vi "Get Dependent Modules.vi"(8 "error in (no error)":errorcluster, 11 "Routing and Faulting Ref in":T1 format="%.0x") -> (0 "error out":errorcluster, 2 "Dependent Modules":T2(array[cluster]) {"Module Ref" format="%.0x"}, 3 "Routing and Faulting Ref out":T1 format="%.0x")   [LabVIEW 2017, in "Routing and Faulting System Explorer.lvlib"]
uses:
  Routing and Faulting System Explorer.lvlib
  <vilib>/NI Veristand/Custom Device API/Custom Device Item Ref.ctl
  <vilib>/NI Veristand/Custom Device API/Get Item Property (String Array).vi
  <vilib>/NI Veristand/Custom Device API/Get Item Property (Dependent Node Pointer).vi
  <vilib>/NI Veristand/Custom Device API/Custom Device API.lvlib
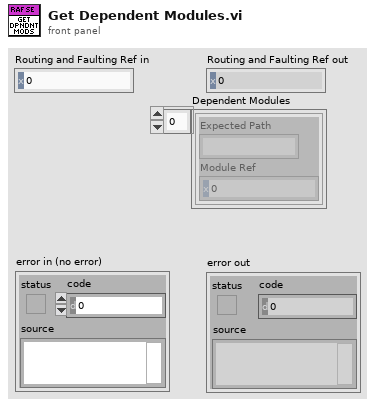
[diagram p1: front panel]
types:
  T1 = typedef "Custom Device API.lvlib/Custom Device Item Ref.ctl" = u64
  T2 = cluster{"Expected Path":string, "Module Ref":T1}[]
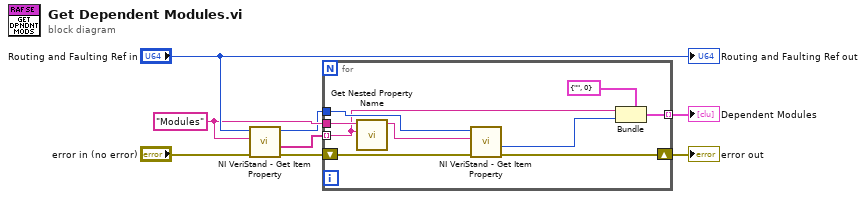
[diagram p0: block diagram]
diagram:
  w5 = "Modules" ("string")
  n1 = call-poly <vilib>:"NI VeriStand - Get Item Property.vi"("error in (no error)"="error in (no error)", "Property Name"=w5, "Item Ref in"="Routing and Faulting Ref in") -> ("error out"=w4:errorcluster, "Value"=w2:string[], "Item Ref out"=w3:T1)  [unwired: 5 in, 1 out]
  n2 = for {
    tunnel: w5 -> [w15]
    shift-right: [w16] -> w7
    shift-left: w4 -> [w14]
    tunnel: w3 -> [w13]
    tunnel: w2 -> [w11] mode=indexing
    tunnel: [w9] -> w1 mode=indexing
    n3 = call "Get Nested Property Name.vi"("property key name"=w11, "property base name"=w15) -> ("full property name"=w17:string)  [unwired: 9 in]
    n4 = call-poly <vilib>:"NI VeriStand - Get Item Property.vi"("error in (no error)"=w14, "Property Name"=w17, "Item Ref in"=w13) -> ("error out"=w16:errorcluster, "Dependent Node Ref"=w10:T1)  [unwired: 5 in, 2 out]
    n5 = Bundle(cluster=cluster{"Expected Path":string, "Module Ref":T1} {"Expected Path"="", "Module Ref"=0} ("Cluster"), "Expected Path"=w11, "Module Ref"=w10) -> (w9:cluster{"Expected Path":string, "Module Ref":T1})
  }
  "error out" <- w7
  "Dependent Modules" <- w1
  "Routing and Faulting Ref out" <- "Routing and Faulting Ref in"
